vi "2 angle_diff_c.vi"   [LabVIEW 2011]
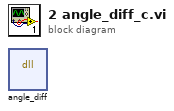
[diagram p0: block diagram]
diagram:
  n1 = dll-call lib="?" fn="angle_diff"() -> ()  [unwired: 8 in, 2 out]
